vi "Commit NVMEM Areas.vi"(8 "error in (no error)":errorcluster, 10 "NVMEM areas":refnum<k21>="$DefaultNVMEMAreas", 11 "SLSC Interface in":refnum<class "SLSC Interface.lvclass">) -> (0 "error out":errorcluster, 3 "SLSC Interface out":refnum<class "SLSC Interface.lvclass">)   [LabVIEW 2015, in "SLSC Interface.lvclass"]
uses:
  SLSC Interface.lvclass
  nvmem type.ctl
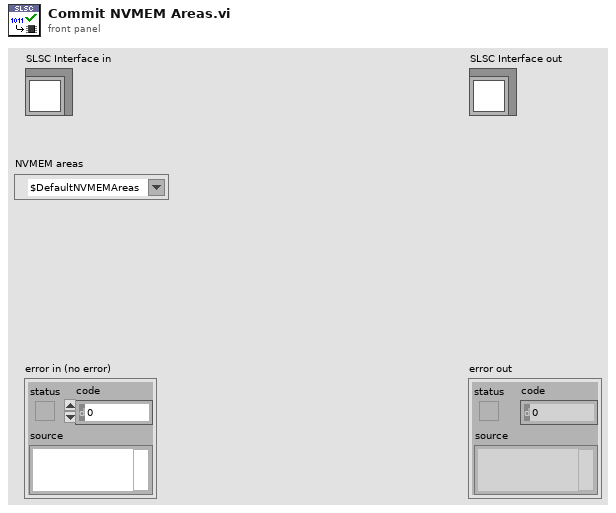
[diagram p1: front panel]
types:
  T1 = typedef "SLSC Interface.lvclass/nvmem type.ctl" = enum16{"area", "device", "session"}
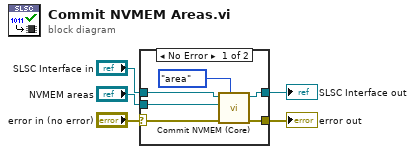
[diagram p0: block diagram]
diagram:
  n1 = case shown="No Error" "error in (no error)" {
    selector: "error in (no error)" -> [w7 w13]
    tunnel: [w6 w13] -> w4
    tunnel: [w8 w12] -> w2
    tunnel: "SLSC Interface in" -> [w11 w12]
    tunnel: "NVMEM areas" -> [w10 _]
    frame No Error {
      n2 = call-dynamic "Commit NVMEM (Core).vi"("nvmem type"=nvmem_type."area", "error in (no error)"=w7, "resources"=w10, "SLSC Interface in"=w11) -> ("error out"=w6:errorcluster, "SLSC Interface out"=w8:refnum<class "SLSC Interface.lvclass">)  [unwired: 6 in]
    }
    frame Error {
    }
  }
  "error out" <- w4
  "SLSC Interface out" <- w2
